vi "Shared Library Path.vi"(8 "error in (no error)":errorcluster) -> (0 "error out":errorcluster, 3 "Path":path)   [LabVIEW 2020, in "LINX API.lvclass"]
uses:
  LINX API.lvclass
  LINX API.lvclass/LINX API.ctl
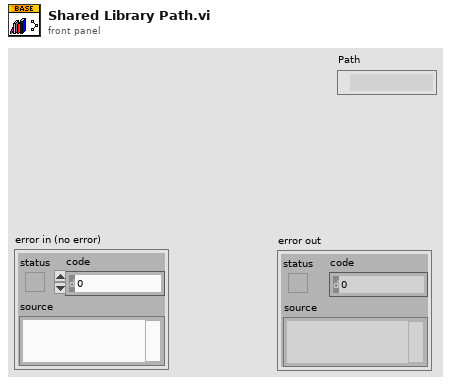
[diagram p1: front panel]
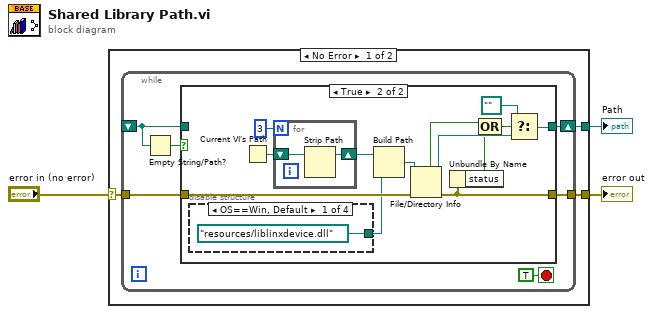
[diagram p0: block diagram]
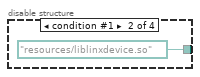
[diagram p3: hidden frame]
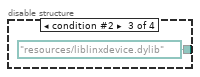
[diagram p4: hidden frame]
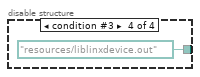
[diagram p5: hidden frame]
diagram:
  n1 = case shown="No Error" "error in (no error)" {
    selector: "error in (no error)" -> [w6 w34]
    tunnel: [w5 _] -> w2
    tunnel: [w4 w34] -> w1
    frame No Error {
      n2 = while {
        shift-right: [w9] -> w5
        shift-left: _ -> [w11]
        tunnel: w6 -> [w10]
        tunnel: [w7] -> w4
        stop <- TRUE stop-if-true
        n3 = Empty String/Path?(string/path=w11) -> (empty?=w12:bool)
        n4 = case shown="True" w12 {
          tunnel: w11 -> [w14 _]
          tunnel: w10 -> [w13 w26]
          tunnel: [w14 w17] -> w9
          tunnel: [w13 w22] -> w7
          frame False {
          }
          frame True {
            n5 = disable-structure shown="OS==Win, Default" {
              disable-tunnel: [path "resources/liblinxdevice.dll" path "resources/liblinxdevice.so" path "resources/liblinxdevice.dylib" path "resources/liblinxdevice.out"] -> w16
              frame condition #0 (active) {
              }
              frame condition #1 {
              }
              frame condition #2 {
              }
              frame condition #3 {
              }
            }
            n6 = Current VI's Path() -> (path=w27:path)
            n7 = for {
              N: 3 -> [_]
              shift-right: [w32] -> w24
              shift-left: w27 -> [w33]
              n8 = Strip Path(path=w33) -> (stripped path=w32:path)  [unwired: 1 out]
            }
            n9 = Build Path(base path=w24, name or relative path=w16) -> (appended path=w23:path)
            n10 = File/Directory Info(path=w23, error in=w26) -> (path out=w21:path, directory=w20:bool, error out=w22:errorcluster)  [unwired: 4 out]
            n11 = Unbundle By Name(w22) -> ("status"=w19:bool)
            n12 = Compound Arithmetic op=OR(w20, w19) -> (w18:bool)
            n13 = Select(t=path "", s=w18, f=w21) -> (s? t:f=w17:path)
          }
        }
      }
    }
    frame Error {
    }
  }
  "Path" <- w2
  "error out" <- w1
